vi "Do Critical Stuff.vi"() -> ()   [LabVIEW 2017]
uses:
  <vilib>/userdefined/High Color/nirio_resource_hc.ctl
  <vilib>/LabVIEW Targets/FPGA/cRIO/shared/nicrio_ModuleControls/nicrio_cRIO-9232_ConfigModeRing.ctl
  <vilib>/LabVIEW Targets/FPGA/cRIO/shared/nicrio_ModuleControls/nicrio_cRIO-9230_DataRatesRing2.ctl
  <vilib>/LabVIEW Targets/FPGA/cRIO/shared/nicrio_ModuleControls/nicrio_cRIO-9227_DataRatesRing.ctl
  <vilib>/Platform/TimedLoop/XDataNode/timing_clust.ctl
  <vilib>/Platform/TimedLoop/XDataNode/nitl_modes.ctl
  <vilib>/Platform/TimedLoop/XDataNode/wakeup.ctl
  <vilib>/FPGAPlugInAG/cRIO-9035/niLvFpga_Open_cRIO-9035.vi
  <vilib>/rvi/interface/common/dynamic/niFpgaDynamicAddResources.vi
  <vilib>/FPGAPlugInAG/Dynamic/niLvFpga_Reset_Dynamic.vi
  <vilib>/Utility/error.llb/Error Cluster From Error Code.vi
  <vilib>/rvi/errors/niLvFpgaAdjustHostInterfaceError.vi
  <vilib>/FPGAPlugInAG/Dynamic/niLvFpga_Run_Dynamic.vi
  <vilib>/RVI Host/nirviSupport.llb/nirviErrorClusterFromErrorCode.vi
  <vilib>/LabVIEW Targets/FPGA/RIO/CompactRIO/cRIO-91xx/cRIO-91XX_ReadTEDSImpl.vi
  <vilib>/FPGAPlugInAG/cRIO-9035/niLvFpga_Reset_cRIO-9035.vi
  <vilib>/FPGAPlugInAG/cRIO-9035/niLvFpga_Run_cRIO-9035.vi
  <vilib>/Platform/TimedLoop/XDataNode/loadnilvce.vi
  <vilib>/FPGAPlugInAG/cRIO-9035/niLvFpga_Close_cRIO-9035.vi
  <vilib>/FPGAPlugInAG/Dynamic/niLvFpga_Close_Dynamic.vi
  <vilib>/rvi/interface/nirviOpenFPGA/nirviOpenFPGA.xnode
  FPGA Bitfiles/80Ton_FPGATarget_accelerometer_vQr4SS40msc.lvbitx
  FPGA Bitfiles/accelerometer.vi
  <vilib>/rvi/interface/nirviMethod/nirviMethod.xnode
  <vilib>/rvi/interface/nirviReadWriteControl/nirviReadWriteControl.xnode
  <vilib>/platform/TimedLoop/XDataNode/XDataNode.xnode
  <vilib>/rvi/interface/nirviCloseFPGA/nirviCloseFPGA.xnode
  <vilib>/rvi/interface/nirviMethod/StockFPGA_InlinedMethodWaitForSingleIRQ.vi
  <vilib>/FPGAPlugInAG/Dynamic/niLvFpga_WaitOnIrq_Dynamic.vi
  <vilib>/FPGAPlugInAG/Dynamic/niLvFpga_AcknowledgeIrq_Dynamic.vi
  NiFpgaLv.dll
  <vilib>/rvi/interface/Simulation/niFpgaSimulationCallBeginRW.vi
  <vilib>/Platform/TimedLoop/XDataNode/XDNodeRunTimeDep.lvlib
panel:
  out "Compressor VFD Output Current (A)":dbl
  out "Compressor VFD Output Frequency (Hz)":dbl
  out "Water Pump Frequency (Hz)":dbl
  in  "Are the values not stupid numbers anymore?":bool
  out "Host error out 2":errorcluster
  out "FPGA error out":errorcluster
  out "Elements Remaining 2":u32
  out "Data FIFO Full 2":bool
  in  "Full Open Time":dbl
  out "Waveform Graph 3":dbl[](graph)
  out "loop iter":i32
  out "loopcheck":i32
  out "millisecond timer value 3":u32
  out "millisecond timer value 4":u32
  out "loopcheck 2":i32
  out "100% Open Time 2":dbl
  out "millisecond timer value 5":u32
  out "millisecond timer value 6":u32
  out "millisecond timer value 8":u32
  out "millisecond timer value 7":u32
  out "%oOpen_save":dbl format="%#_13g"
  out "size(s)":i32
  in  "?":bool
  out "Pdis2":dbl
  in  "output cluster":T1
  out "loop iter 4":u32
  out "loop iter 3":u32
  in  "Economizer ?":bool
  out "loop iter 2":i32
  out "x > y?":bool
  out "x .and. y?":bool
  out "Host error out 3":errorcluster
  out "result":bool
  out "FPGA Error Out":errorcluster
  out "Host error out":errorcluster
  in  "Host Loop update rate (ms)":u32=100
  in  "stop":bool
  out "Elements Remaining":u32
  out "Open Loop":bool[](array[boolean])
  out "Short Circuit":bool[](array[boolean])
  out "Data FIFO Full":bool
  out "Waveform Graph":waveform(dbl)[](graph)
  out "Atmospheric Pressure":dbl
  out "element":dbl
  in  "Path 10":path
  in  "Path 9":path
  in  "Path 8":path
  in  "Path 7":path
  in  "Path 6":path
  in  "Path 5":path
  in  "Path 4":path
  in  "Path":path
  in  "Path 2":path
  in  "Path 3":path
  in  "Tab Control":T2(tab)
  in  "Units":string(combo)="IP"
  in  "?":dbl=0.9992
  in  "Tdis":dbl=0.0747
  in  "?":dbl=-0.0246
  in  "Tsuc":dbl=0.998
  in  "?":dbl
  in  "T07":dbl=1.0
  in  "?":dbl=-0.0404
  in  "Tsuc2":dbl=0.9934
  in  "?":dbl=0.0059
  in  "T05":dbl=0.9998
  in  "?":dbl=0.0161
  in  "T04":dbl=1.0002
  in  "?":dbl=0.0174
  in  "Tdis2":dbl=0.9998
  in  "P03":dbl=0.9962
  in  "?":dbl=0.0158
  in  "P04":dbl=0.9943
  in  "?":dbl=-0.8769
  in  "P01":dbl=1.0
  in  "?":dbl
  in  "P02":dbl=1.0
  in  "?":dbl
  in  "P05":dbl=0.9959
  in  "?":dbl=-0.6009
  in  "P06":dbl=0.991
  in  "?":dbl=-0.236
  in  "P07":dbl=1.0
  in  "?":dbl
  in  "P08":dbl=0.9971
  in  "?":dbl=-0.509
  in  "P09":dbl=0.9954
  in  "?":dbl=-0.7109
  in  "Controller Toggle P 2":bool
  in  "Reinitialize Controller P 2":bool
  in  "Current Intermediate P":dbl format="%#_13g"
  in  "Desired Intermediate P":dbl
  in  "Controller Toggle T 2":bool
  in  "Reinitialize Controller T 2":bool
  in  "Current Intermediate T":dbl format="%#_13g"
  in  "Desired Intermediate T":dbl
  in  "?":enum32{"Page 1", "Page 2"}(tab)
  out "Economizer\nFine Liquid Position":dbl(slide) min=0.0 max=100.0 step=1.0 scale=0.0..100.0
  in  "Economizer\nFine Liquid Adjust":dbl(slide) min=0.0 max=100.0 step=1.0 scale=0.0..100.0
  out "Economizer\nLiquid Coarse Position":dbl(slide) min=0.0 max=100.0 step=1.0 scale=0.0..100.0
  in  "Economizer\nLiquid Coarse Adjust":dbl(slide) min=0.0 max=100.0 step=1.0 scale=0.0..100.0
  in  "PID gains in Coarse Liquid":T3
  in  "PID gains in Fine Liquid":T3
  in  "Autotune CoarseLiquid":bool
  in  "Accept Autotune Coarse Liquid":bool
  in  "Autotune Fine Liquid":bool
  in  "Accept Autotune Fine Liquid":bool
  out "PID gains out Coarse Liquid":T3
  out "PID gains out Fine Liquid":T3
  out "tuning completed? Coarse Liquid":bool
  out "tuning completed? Fine Liquid":bool
  in  "?":enum32{"Page 1", "Page 2"}(tab)
  out "Economizer Gas\n Fine Position":dbl(slide) min=0.0 max=100.0 step=1.0 scale=0.0..100.0
  in  "Economizer Gas\n Fine Adjust":dbl(slide) min=0.0 max=100.0 step=1.0 scale=0.0..100.0
  out "Economizer Gas\n Coarse Position":dbl(slide) min=0.0 max=100.0 step=1.0 scale=0.0..100.0
  in  "Economizer Gas\n Coarse Adjust":dbl(slide) min=0.0 max=100.0 step=1.0 scale=0.0..100.0
  in  "PID gains in Coarse gas":T3
  in  "PID gains in Fine Gas":T3
  in  "Autotune Coarse":bool
  in  "Accept Autotune Coarse":bool
  in  "Autotune Fine Gas":bool
  in  "Accept Autotune Fine":bool
  out "PID gains out Coarse Gas":T3
  out "PID gains out Fine Gas":T3
  out "tuning completed? Coarse Gas":bool
  out "tuning completed? Fine Gas":bool
  in  "?":bool
  in  "Reinitialize Controller T":bool
  in  "Delta T Threshold":dbl=5.0 format="%#_13g"
  in  "Tonnage Threshold":dbl=40.0 format="%#_13g"
  in  "Delta P Threshold":dbl=5.0 format="%#_13g"
  in  "Desired Tsuc":dbl
  in  "Desired Psuc":dbl
  in  "Tab Control 3":enum32{"Page 1", "Page 2", "Page 3"}(tab)
  in  "Small Liquid Adjust":dbl(slide) scale=0.0..100.0 scale format="%#_3g"
  in  "Medium Liquid Adjust":dbl(slide) scale=0.0..100.0 scale format="%#_3g"
  in  "Large Liquid Adjust  2":dbl(slide) scale=0.0..100.0 scale format="%#_3g"
  out "Output Large Liq":dbl(slide) scale=0.0..100.0
  out "Output Medium Liq":dbl(slide) scale=0.0..100.0
  out "Output Small Liq":dbl(slide) scale=0.0..100.0
  in  "Accept Autotune Small Liquid":bool
  in  "Autotune Small Liquid":bool
  in  "PID gains in Small Liquid":T3={"proportional gain (Kc)"=-0.0413, "integral time (Ti, min)"=12.063, "derivative time (Td, min)"=0.0}
  in  "PID gains in Medium Liquid":T3={"proportional gain (Kc)"=-0.22, "integral time (Ti, min)"=2.9, "derivative time (Td, min)"=0.0}
  in  "Accept Autotune Medium Liquid":bool
  in  "Autotune Medium Liquid":bool
  in  "PID gains in Large Liquid":T3
  in  "Accept Autotune Large  Liquid":bool
  in  "Autotune Large Liquid":bool
  out "PID gains out Large Liquid":T3
  out "PID gains out Medium Liquid":T3
  out "PID gains out Small Liquid":T3
  out "tuning completed? Large Liq":bool
  out "tuning completed? Medium Liq":bool
  out "tuning completed? Small Liq":bool
  out "Suction Temperature":dbl[][](graph)
  in  "Tab Control 2":enum32{"Page 1", "Page 2", "Page 3"}(tab)
  in  "Large Gas Adjust":dbl(slide) scale=0.0..100.0 scale format="%#_3g"
  in  "Medium Gas Adjust":dbl(slide) scale=0.0..100.0 scale format="%#_3g"
  in  "Small Gas Adjust":dbl(slide) scale=0.0..100.0 scale format="%#_3g"
  out "Output Large Gas":dbl(slide) scale=0.0..100.0
  out "Output Medium Gas":dbl(slide) scale=0.0..100.0
  out "Output Small Gas":dbl(slide) scale=0.0..100.0
  in  "PID gains in Large gas":T3
  in  "PID gains in Medium Gas":T3={"proportional gain (Kc)"=0.542, "integral time (Ti, min)"=2.03, "derivative time (Td, min)"=0.0}
  in  "PID gains in Small Gas":T3={"proportional gain (Kc)"=0.173, "integral time (Ti, min)"=0.636, "derivative time (Td, min)"=0.0}
  in  "Autotune Large":bool
  in  "Accept Autotune Large":bool
  in  "Autotune Medium Gas":bool
  in  "Accept Autotune Medium":bool
  in  "Autotune Small":bool
  in  "Accept Autotune Small":bool
  out "PID gains out Large Gas":T3
  out "PID gains out Medium Gas":T3
  out "PID gains out Small Gas":T3
  out "tuning completed? Large Gas":bool
  out "tuning completed? Medium Gas":bool
  out "tuning completed? Small Gas":bool
  out "Suction Pressure":dbl[][](graph)
  in  "Reinitialize Controller P":bool
  in  "?":bool
  out "Controller Toggle T":bool
  out "Controller Toggle P":bool
  out "Current Tsuc":dbl format="%#.3g"
  out "Current Psuc":dbl format="%#.3g"
  out "Controller Toggle T 3":bool
  out "Controller Toggle P 3":bool
  out "Pdis":dbl format="%#.3g"
  out "element 2":dbl
  out "Tonnage":dbl
  in  "file for water pump 2":path
  in  "Fine slide in P 3":refnum<vi>
  in  "?":enum32{"Page 1", "Page 2", "Page 3"}(tab)
  in  "Coarse Water Adjust":dbl(slide) scale=0.0..100.0 scale format="%#_3g"
  out "Water Valve Output":dbl(slide) scale=0.0..100.0 scale format="%#_3g"
  in  "Fine Water Adjust":dbl(slide) scale=0.0..60.0 scale format="%#_3g"
  out "Water Pump Output":dbl(slide) scale=0.0..60.0 scale format="%#_3g"
  in  "PID gains in Water Valve":T3={"proportional gain (Kc)"=0.081, "integral time (Ti, min)"=6.75, "derivative time (Td, min)"=0.0}
  out "PID gains out Coarse Water":T3
  in  "autotune? Coarse Water":bool
  in  "Accept Autotune Water":bool
  out "tuning completed? Water Valve":bool
  in  "PID gains in water pump 2":T3={"proportional gain (Kc)"=-0.161, "integral time (Ti, min)"=1.936, "derivative time (Td, min)"=0.0}
  out "PID gains out (fine water)":T3
  in  "autotune? water pump 2":bool
  in  "Accept Autotune Water Pump 2":bool
  out "tuning completed? Water Pump":bool
  out "Discharge Pressure":dbl[][](graph)
  in  "file for fine gas":path
  in  "Fine slide in P 2":refnum<vi>
  in  "Desired Pdis":dbl
  in  "Reinitialize Controller":bool
  in  "Controller Toggle P 4":bool
  out "Controller Toggle Water":bool
  in  "Condensing Press Threshold":dbl=5.0 format="%#_13g"
  out "Current Pdis":dbl format="%#.3g"
  in  "Start Water Pump":bool
  in  "Tab Control 4":enum32{"Page 1", "Page 2"}(tab)
  in  "Oil Pump Speed Adjust":dbl(slide) min=0.0 max=100.0 step=1.0 scale=0.0..60.0
  out "Oil Pump Output":dbl(slide) scale=0.0..60.0
  in  "PID gains in oil pump":T3
  out "PID gains out oil pump":T3
  in  "autotune? oil pump":bool
  in  "Accept Autotune Oil Pump":bool
  out "tuning completed?":bool
  in  "Start Oil Pump":bool
  out "Closed":bool
  out "Open":bool
  in  "Timing Complete?":bool
  in  "Open":bool
  in  "Close":bool
  in  "Close 2":bool
  in  "Open 2":bool
  in  "RIO Device 2":T4="RIO0"
  in  "Data Rate 2":T5=25 items=["50.000 kS/s (NI 9227)"=1, "25.000 kS/s (NI 9227)"=2, "16.667 kS/s (NI 9227)"=3, "12.500 kS/s (NI 9227)"=4, "10.000 kS/s (NI 9227)"=5, "8.333 kS/s (NI 9227)"=6, "7.143 kS/s (NI 9227)"=7, "6.250 kS/s (NI 9227)"=8, "5.556 kS/s (NI 9227)"=9, "5.000 kS/s (NI 9227)"=10, "4.545 kS/s (NI 9227)"=11, "4.167 kS/s (NI 9227)"=12, "3.846 kS/s (NI 9227)"=13, "3.571 kS/s (NI 9227)"=14, "3.333 kS/s (NI 9227)"=15, "3.125 kS/s (NI 9227)"=16, "2.941 kS/s (NI 9227)"=17, "2.778 kS/s (NI 9227)"=18, "2.632 kS/s (NI 9227)"=19, "2.500 kS/s (NI 9227)"=20, "2.381 kS/s (NI 9227)"=21, "2.273 kS/s (NI 9227)"=22, "2.174 kS/s (NI 9227)"=23, "2.083 kS/s (NI 9227)"=24, "2.000 kS/s (NI 9227)"=25, "1.923 kS/s (NI 9227)"=26, "1.852 kS/s (NI 9227)"=27, "1.786 kS/s (NI 9227)"=28, "1.724 kS/s (NI 9227)"=29, "1.667 kS/s (NI 9227)"=30, "1.613 kS/s (NI 9227)"=31]
  in  "Host Loop update rate (ms) 2":u32=100
  out "Waveform Graph 2":waveform(dbl)[](graph)
  in  "stop 2":bool
  out "millisecond timer value":u32
  out "100% Open Time":dbl
  out "millisecond timer value 2":u32
  out "%Open":dbl(slide) scale=0.0..100.0
  out "Closed 2":bool
  out "Open  3":bool
  out "Controller Toggle Oil Pump":bool
  in  "Controller Toggle P 8":bool
  in  "Fine slide in P 4":refnum<vi>
  in  "file for oil pump 3":path
  in  "PID gains in water pump":T3
  in  "autotune? water pump":bool
  in  "file for water pump":path
  in  "Fine slide in P":refnum<vi>
  in  "Accept Autotune Water Pump":bool
  in  "Compressor Speed Adjust":dbl(slide) min=0.0 max=100.0 step=1.0 scale=0.0..60.0
  in  "Controller Toggle P 6":bool=TRUE
  out "acceleration v time":waveform(dbl)[](graph)
  in  "RIO Device":T4="RIO0"
  in  "Display TEDS Data":bool
  in  "TEDS Template File Directory":path=path "C:/"
  in  "Input Configuration":T6=2 items=["AC Coupled", "DC Coupled", "IEPE AC Coupled"]
  in  "Data Rate":T7=10 items=["12.800 kS/s (NI 9230)"=10, "11.378 kS/s (NI 9230)"=36, "10.240 kS/s (NI 9230)"=21, "9.309 kS/s (NI 9230)"=44, "8.533 kS/s (NI 9230)"=14, "7.877 kS/s (NI 9230)"=52, "7.314 kS/s (NI 9230)"=29, "6.827 kS/s (NI 9230)"=60, "6.400 kS/s (NI 9230)"=18, "6.024 kS/s (NI 9230)"=68, "5.689 kS/s (NI 9230)"=37, "5.389 kS/s (NI 9230)"=76, "5.120 kS/s (NI 9230)"=22, "4.876 kS/s (NI 9230)"=84, "4.655 kS/s (NI 9230)"=45, "4.452 kS/s (NI 9230)"=92, "4.267 kS/s (NI 9230)"=26, "4.096 kS/s (NI 9230)"=100, "3.938 kS/s (NI 9230)"=53, "3.657 kS/s (NI 9230)"=30, "3.413 kS/s (NI 9230)"=61, "3.200 kS/s (NI 9230)"=34, "3.012 kS/s (NI 9230)"=69, "2.844 kS/s (NI 9230)"=38, "2.695 kS/s (NI 9230)"=77, "2.560 kS/s (NI 9230)"=42, "2.438 kS/s (NI 9230)"=85, "2.327 kS/s (NI 9230)"=46, "2.226 kS/s (NI 9230)"=93, "2.133 kS/s (NI 9230)"=50, "2.048 kS/s (NI 9230)"=101, "1.969 kS/s (NI 9230)"=54, "1.829 kS/s (NI 9230)"=58, "1.707 kS/s (NI 9230)"=62, "1.600 kS/s (NI 9230)"=66, "1.506 kS/s (NI 9230)"=70, "1.422 kS/s (NI 9230)"=74, "1.347 kS/s (NI 9230)"=78, "1.280 kS/s (NI 9230)"=82, "1.219 kS/s (NI 9230)"=86, "1.164 kS/s (NI 9230)"=90, "1.113 kS/s (NI 9230)"=94, "1.067 kS/s (NI 9230)"=98, "1.024 kS/s (NI 9230)"=102, "0.985 kS/s (NI 9230)"=106]
  out "magnitudes":cluster{"f0":dbl, "df":dbl, "magnitude":dbl[]}[](graph)
  out "rotational speed (rpm)":dbl
  out "Compressor Speed (Hz)":dbl
  out "Controller Toggle P 5":bool
  out "Compressor Speed Output":dbl(slide) scale=0.0..60.0
  in  "Start Compressor":bool
  out "Spool x acceleration (Hz)":dbl
  out "Spool y acceleration (Hz)":dbl
  # "Thermocouple Calibration Data"
  # "Pressure Transducer Calibration Data"
  # "Slope"
  # "y-intercept"
  # "Slope"
  # "y-intercept"
  # "Start Up Procedure"
  # "1. Check all safety circuit components to make sure safety loop is closed and VFD's have no faults\n\n2. Check that suction and discharge ball valves are in the open position\n\n3. Put EXV and Oil valves into position\n\n4. Check oil separator sight glass for oil\n\n5. Start cooling water\n\n6. Start compressor"
  # "RTD Calibration Data"
  # "Slope"
  # "y-intercept"
  # "Coarse Water Adjust - Valve"
  # "Fine Water Adjust - Pump"
  # "Oil Pump Speed Control"
  # "Compressor Speed Control"
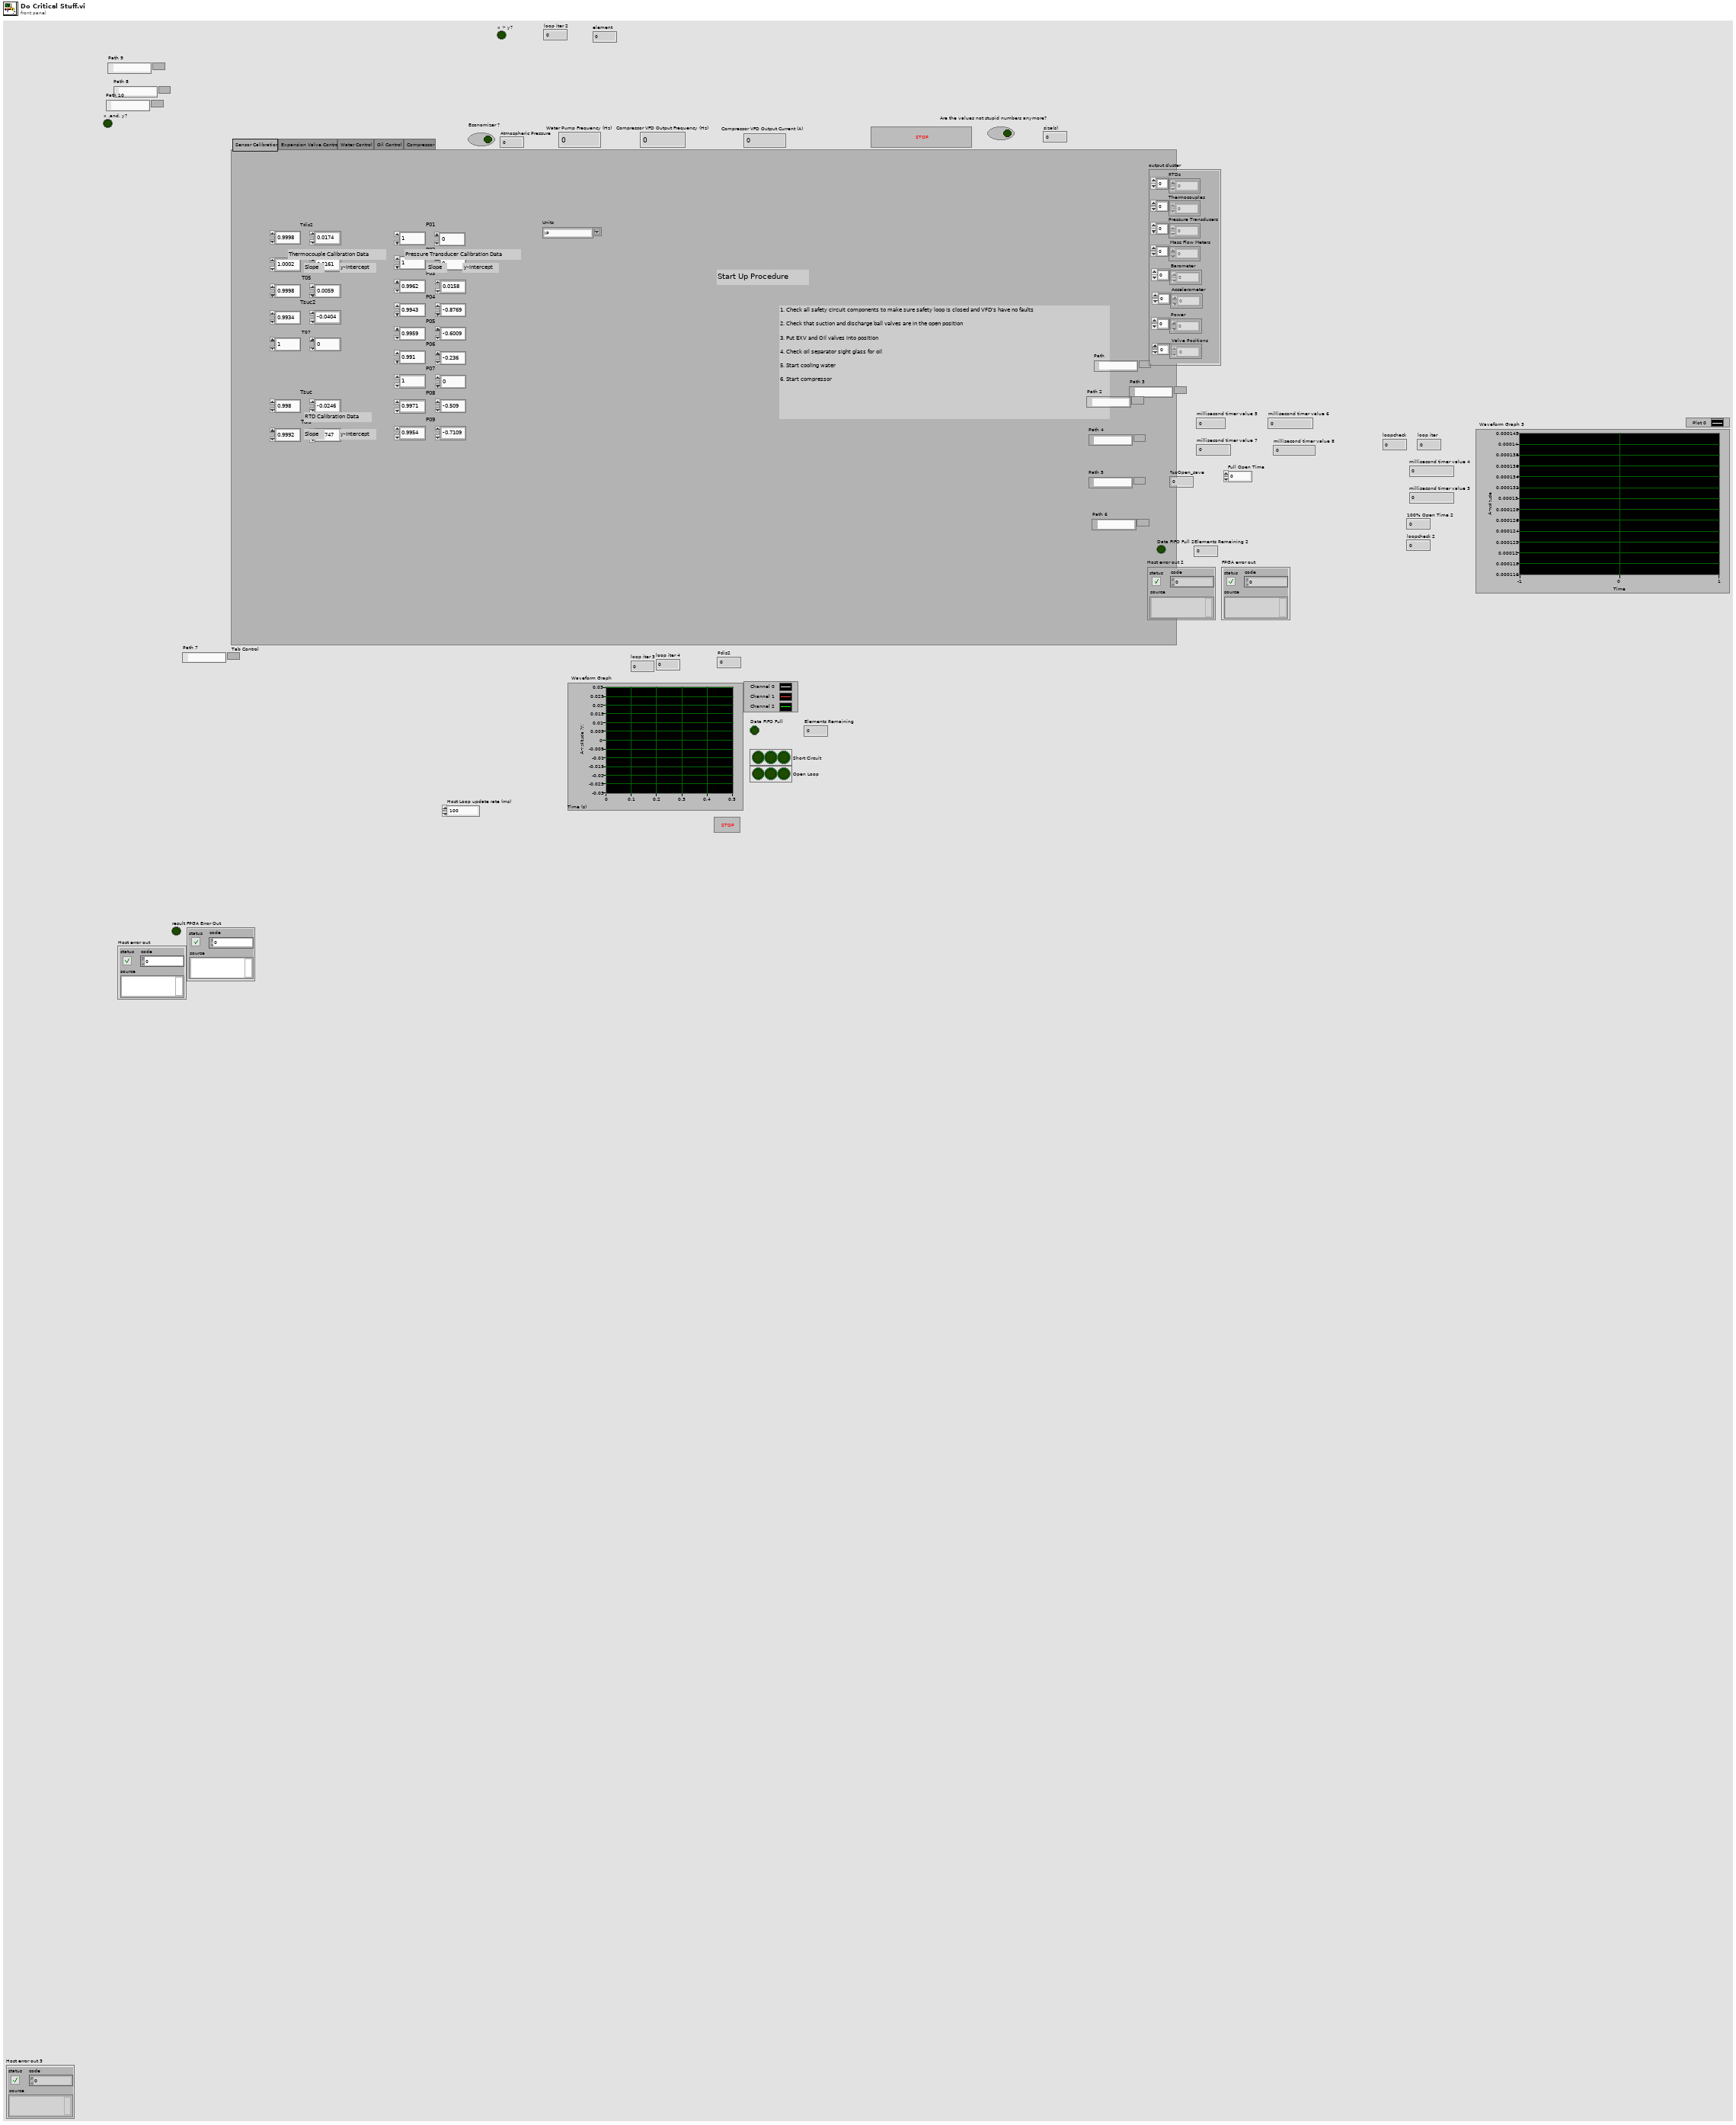
[diagram p1: front panel]
types:
  T1 = cluster{"RTDs":dbl[], "Thermocouples":dbl[], "Pressure Transducers":dbl[], "Mass Flow Meters":dbl[], "Barometer":dbl[], "Accelerometer":dbl[], "Power":dbl[], "Valve Positions":dbl[]}
  T2 = enum32{"Sensor Calibration", "Expansion Valve Control", "Water Control", "Oil Control", "Compressor"}
  T3 = cluster{"proportional gain (Kc)":dbl, "integral time (Ti, min)":dbl, "derivative time (Td, min)":dbl}
  T4 = typedef "nirio_resource_hc.ctl" = tag
  T5 = typedef "nicrio_cRIO-9227_DataRatesRing.ctl" = u8
  T6 = typedef "nicrio_cRIO-9232_ConfigModeRing.ctl" = u8
  T7 = typedef "nicrio_cRIO-9230_DataRatesRing2.ctl" = u8
  T8 = cluster{"TEDS Error?":bool, "TEDS Error":string, "TEDS Data":string[][]}
  T9 = typedef "XDNodeRunTimeDep.lvlib/timing_clust.ctl" = cluster{"Expected End [f-1]":u64, "Actual End [f-1]":u64, "Finished Late? [f-1]":bool, "Expected End [i-1]":u64, "Actual End [i-1]":u64, "Finished Late? [i-1]":bool, "Expected Start [i]":u64, "Actual Start [i]":u64, "Expected Start [f]":u64, "Actual Start [f]":u64, "Source Name":string, "Structure Name":string, "Period":i64, "Deadline":i64, "Offset":i64, "Start":i64, "Priority":i32, "Timeout":i32, "Mode":T10, "Wakeup Reason":T11, "Error":errorcluster, "Source Type":string, "Secondary Source Type":string, "Global End Time":u64, "Global Start Time":u64, "Frame Duration":u64, "Iteration Duration":u64, "Assigned CPU":i32, "I/O Scan Engine Mode":u32}
  T10 = typedef "XDNodeRunTimeDep.lvlib/nitl_modes.ctl" = enum32{"No Change", "Process missed periods, maintain original phase", "Discard missed periods, maintain original phase", "Process missed periods, ignore original phase", "Discard missed periods, ignore original phase"}
  T11 = typedef "XDNodeRunTimeDep.lvlib/wakeup.ctl" = enum32{"Normal", "Aborted", "Asynchronous wakeup", "Timing source error", "Timed loop error", "Timeout"}
  T12 = cluster{"Compressor Speed Adjust":dbl, "autotune? water pump":bool, "Fine slide in P":refnum<vi>, "file for water pump":path, "Accept Autotune Water Pump":bool, "PID gains in water pump":cluster{"proportional gain (Kc)":dbl, "integral time (Ti, min)":dbl, "derivative time (Td, min)":dbl}}
  T13 = cluster{"Oil Pump Speed Adjust":dbl, "autotune? oil pump ":bool, "Fine slide in P 4":refnum<vi>, "file for oil pump 3":path, "Accept Autotune Oil Pump":bool, "PID gains in oil pump ":cluster{"proportional gain (Kc)":dbl, "integral time (Ti, min)":dbl, "derivative time (Td, min)":dbl}}
  T14 = cluster{"output to slide":dbl, "PID gains out":cluster{"proportional gain (Kc)":dbl, "integral time (Ti, min)":dbl, "derivative time (Td, min)":dbl}, "tuning completed?":bool, "Controller Toggle P 2":bool}
  T15 = cluster{"Coarse Water Adjust":dbl, "autotune? Coarse Water":bool, "Fine slide in P 2":refnum<vi>, "file for fine gas":path, "Accept Autotune Water":bool, "PID gains in Water Valve":cluster{"proportional gain (Kc)":dbl, "integral time (Ti, min)":dbl, "derivative time (Td, min)":dbl}}
  T16 = cluster{"Fine Water Adjust":dbl, "autotune? water pump 2":bool, "Fine slide in P 3":refnum<vi>, "file for water pump 2":path, "Accept Autotune Water Pump 2":bool, "PID gains in water pump 2":cluster{"proportional gain (Kc)":dbl, "integral time (Ti, min)":dbl, "derivative time (Td, min)":dbl}}
  T17 = cluster{"output to slide":dbl, "PID gains out":cluster{"proportional gain (Kc)":dbl, "integral time (Ti, min)":dbl, "derivative time (Td, min)":dbl}, "tuning completed?":bool, "output to slide":dbl, "PID gains out":cluster{"proportional gain (Kc)":dbl, "integral time (Ti, min)":dbl, "derivative time (Td, min)":dbl}, "tuning completed?":bool, "Controller Toggle P 2":bool, bool}
  T18 = cluster{"Economizer Gas\n Coarse Adjust":dbl, "Accept Autotune Coarse":bool, "Economizer Gas\n Coarse Adjust":refnum<vi>, "Path 7":path, "Autotune Coarse":bool, "PID gains in Coarse gas ":cluster{"proportional gain (Kc)":dbl, "integral time (Ti, min)":dbl, "derivative time (Td, min)":dbl}}
  T19 = cluster{"Economizer Gas\n Fine Adjust":dbl, "Accept Autotune Fine":bool, "Economizer Gas\n Fine Adjust":refnum<vi>, "Path 8":path, "Autotune Fine Gas ":bool, "PID gains in Fine Gas":cluster{"proportional gain (Kc)":dbl, "integral time (Ti, min)":dbl, "derivative time (Td, min)":dbl}}
  T20 = cluster{"Economizer\nLiquid Coarse Adjust":dbl, "Accept Autotune Coarse Liquid":bool, "Economizer\nLiquid Coarse Adjust":refnum<vi>, "Path 9":path, "Autotune CoarseLiquid":bool, "PID gains in Coarse Liquid":cluster{"proportional gain (Kc)":dbl, "integral time (Ti, min)":dbl, "derivative time (Td, min)":dbl}}
  T21 = cluster{"Economizer\nFine Liquid Adjust":dbl, "Accept Autotune Fine Liquid":bool, "Economizer\nFine Liquid Adjust":refnum<vi>, "Path 10":path, "Autotune Fine Liquid":bool, "PID gains in Fine Liquid":cluster{"proportional gain (Kc)":dbl, "integral time (Ti, min)":dbl, "derivative time (Td, min)":dbl}}
  T22 = cluster{"Hot Gas Bypass\n Fine Position":dbl, "PID gains out fine gas":cluster{"proportional gain (Kc)":dbl, "integral time (Ti, min)":dbl, "derivative time (Td, min)":dbl}, "tuning completed? fine gas":bool, "Hot Gas Bypass\n Coarse Position":dbl, "PID gains out coarse gas":cluster{"proportional gain (Kc)":dbl, "integral time (Ti, min)":dbl, "derivative time (Td, min)":dbl}, "tuning completed? coarse gas":bool, "P Indicator":bool}
  T23 = cluster{"Liquid\n Fine Position":dbl, "PID gains out fine liq":cluster{"proportional gain (Kc)":dbl, "integral time (Ti, min)":dbl, "derivative time (Td, min)":dbl}, "tuning completed? fine liq":bool, "Liquid\n Coarse Position":dbl, "PID gains out coarse liq":cluster{"proportional gain (Kc)":dbl, "integral time (Ti, min)":dbl, "derivative time (Td, min)":dbl}, "tuning completed? coarse liq":bool, "T Indicator":bool}
  T24 = cluster{"Large Gas Adjust ":dbl, "Autotune Large":bool, "Path":path, "Large Gas Adjust ":refnum<vi>, "Accept Autotune Large ":bool, "PID gains in Large gas":cluster{"proportional gain (Kc)":dbl, "integral time (Ti, min)":dbl, "derivative time (Td, min)":dbl}}
  T25 = cluster{"Medium Gas Adjust":dbl, "Autotune Medium Gas":bool, "Path 2":path, "Medium Gas Adjust":refnum<vi>, "Accept Autotune Medium":bool, "PID gains in Medium Gas":cluster{"proportional gain (Kc)":dbl, "integral time (Ti, min)":dbl, "derivative time (Td, min)":dbl}}
  T26 = cluster{"Small Gas Adjust":dbl, "Autotune Small":bool, "Path 3":path, "Small Gas Adjust":refnum<vi>, "Accept Autotune Small":bool, "PID gains in Small Gas ":cluster{"proportional gain (Kc)":dbl, "integral time (Ti, min)":dbl, "derivative time (Td, min)":dbl}}
  T27 = cluster{"Large Liquid Adjust  2":dbl, "Autotune Large Liquid":bool, "Path 4":path, "Large Liquid Adjust  2":refnum<vi>, "Accept Autotune Large  Liquid":bool, "PID gains in Large Liquid":cluster{"proportional gain (Kc)":dbl, "integral time (Ti, min)":dbl, "derivative time (Td, min)":dbl}}
  T28 = cluster{"Medium Liquid Adjust":dbl, "Autotune Medium Liquid":bool, "Path 5":path, "Medium Liquid Adjust":refnum<vi>, "Accept Autotune Medium Liquid":bool, "PID gains in Medium Liquid":cluster{"proportional gain (Kc)":dbl, "integral time (Ti, min)":dbl, "derivative time (Td, min)":dbl}}
  T29 = cluster{"Small Liquid Adjust ":dbl, "Autotune Small Liquid":bool, "Path 6":path, "Small Liquid Adjust ":refnum<vi>, "Accept Autotune Small Liquid":bool, "PID gains in Small Liquid":cluster{"proportional gain (Kc)":dbl, "integral time (Ti, min)":dbl, "derivative time (Td, min)":dbl}}
  T30 = cluster{"output to slide":dbl, "PID gains out":cluster{"proportional gain (Kc)":dbl, "integral time (Ti, min)":dbl, "derivative time (Td, min)":dbl}, "tuning completed?":bool, "output to slide":dbl, "PID gains out":cluster{"proportional gain (Kc)":dbl, "integral time (Ti, min)":dbl, "derivative time (Td, min)":dbl}, "tuning completed?":bool, "output to slide":dbl, "PID gains out":cluster{"proportional gain (Kc)":dbl, "integral time (Ti, min)":dbl, "derivative time (Td, min)":dbl}, "tuning completed?":bool, "Controller Toggle P":bool, bool, bool}
  T31 = cluster{"output to slide":dbl, "PID gains out":cluster{"proportional gain (Kc)":dbl, "integral time (Ti, min)":dbl, "derivative time (Td, min)":dbl}, "tuning completed?":bool, "output to slide":dbl, "PID gains out":cluster{"proportional gain (Kc)":dbl, "integral time (Ti, min)":dbl, "derivative time (Td, min)":dbl}, "tuning completed?":bool, "output to slide":dbl, "PID gains out":cluster{"proportional gain (Kc)":dbl, "integral time (Ti, min)":dbl, "derivative time (Td, min)":dbl}, "tuning completed?":bool, "Controller Toggle T":bool, bool, bool}
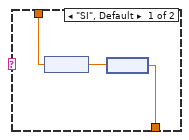
[diagram p5: hidden frame]
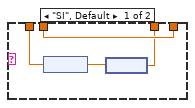
[diagram p6: hidden frame]
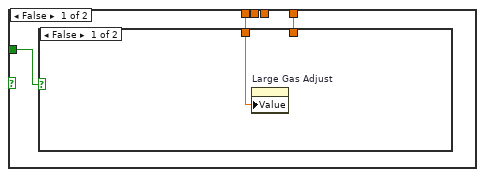
[diagram p8: hidden frame]
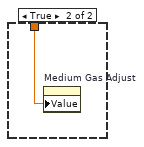
[diagram p9: hidden frame]
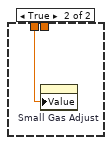
[diagram p10: hidden frame]
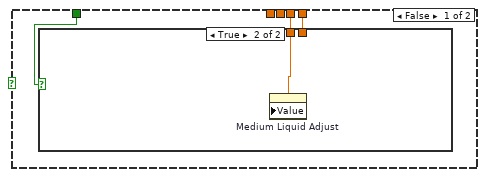
[diagram p12: hidden frame]
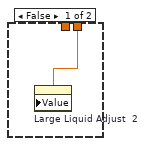
[diagram p13: hidden frame]
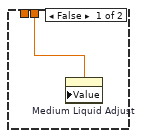
[diagram p14: hidden frame]
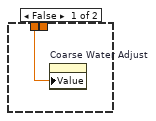
[diagram p16: hidden frame]
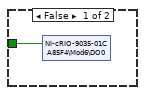
[diagram p19: hidden frame]
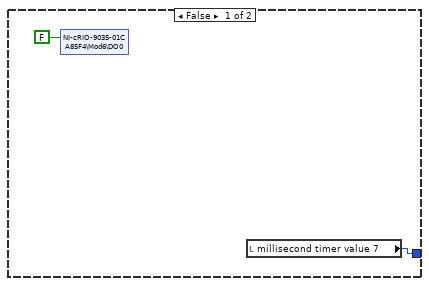
[diagram p20: hidden frame]
diagram:
  w9 = u32 0 ("loop iter 3")
  w10 = u32 0 ("millisecond timer value")
  # "Set up FPGA target"
  n1 = shared-variable "NI-cRIO-9035-01CA85F4\\Untitled Library 2.lvlib\\Data"(dbl[] [] ("Data")) -> ()  [unwired: 1 in, 1 out]
  n2 = xnode "Open FPGA VI Reference"("resource name"="RIO Device") -> ("FPGA VI Reference Out"=w40:refnum<k20>, "error out"=w44:errorcluster)  [unwired: 1 in]
  n3 = xnode "Invoke Method"("FPGA VI Reference In"=w40, "error in"=w44) -> ("FPGA VI Reference Out"=w39:refnum<k20>, "error out"=w41:errorcluster)
  n4 = xnode "Read/Write Control"("FPGA VI Reference In"=w39, "error in"=w41, "Data Rate"="Data Rate", "Input Configuration"="Input Configuration") -> ("FPGA VI Reference Out"=w46:refnum<k20>, "error out"=w45:errorcluster)
  n5 = xnode "Invoke Method"("FPGA VI Reference In"=w46, "error in"=w45) -> ("FPGA VI Reference Out"=w25:refnum<k20>, "error out"=w23:errorcluster)  [unwired: 1 in]
  n6 = xnode "Invoke Method"("FPGA VI Reference In"=w25, "error in"=w23, "IRQ Number(s)"=0, "Timeout (ms)"=15000) -> ("FPGA VI Reference Out"=w24:refnum<k20>, "error out"=w22:errorcluster, "IRQ(s) Asserted"=w16:i32)  [unwired: 1 out]
  n7 = case shown="False" "Display TEDS Data" {
    tunnel: w24 -> [w75 w81]
    tunnel: [w75 w80] -> w18
    tunnel: w22 -> [w74 w79]
    tunnel: [w74 w76] -> w19
    frame False {
    }
    frame True {
      n8 = for {
        N: 3 -> [_]
        tunnel: w81 -> [w92]
        tunnel: [w91] -> w80
        tunnel: [w86] -> w77 mode=indexing
        shift-right: [w87] -> w76
        shift-left: w79 -> [w90]
        i -> [w85]
        n9 = xnode "Invoke Method"("FPGA VI Reference In"=w92, "error in"=w90, "Slot"=1, "Channel"=w85) -> ("FPGA VI Reference Out"=w91:refnum<k20>, "error out"=w88:errorcluster, "TEDS Binary"=w83:bool[], "v0.9 (TEDS)"=w84:bool)
        n10 = call "TEDS Binary to Table.vi"("error in"=w88, "v0.9 TEDS (F)"=w84, "template file directory"="TEDS Template File Directory", "TEDS Binary"=w83) -> ("error out"=w87:errorcluster, "TEDS"=w86:T8)  [unwired: 1 out]
      }
      n11 = call "Display TEDS Data.vi"("TEDS Array"=w77) -> ()  [unwired: 4 out]
    }
  }
  n12 = xnode "Open FPGA VI Reference"("resource name"="RIO Device 2") -> ("FPGA VI Reference Out"=w32:refnum<k20>, "error out"=w29:errorcluster)  [unwired: 1 in]
  n13 = xnode "Invoke Method"("FPGA VI Reference In"=w32, "error in"=w29) -> ("FPGA VI Reference Out"=w31:refnum<k20>, "error out"=w30:errorcluster)
  n14 = local write "%Open"(0.0 ("%Open")) -> ()
  n15 = xnode "Read/Write Control"("FPGA VI Reference In"=w31, "error in"=w30, "Data Rate"="Data Rate 2") -> ("FPGA VI Reference Out"=w27:refnum<k20>, "error out"=w28:errorcluster)
  n16 = xnode "Invoke Method"("FPGA VI Reference In"=w27, "error in"=w28) -> ("FPGA VI Reference Out"=w15:refnum<k20>, "error out"=w7:errorcluster)  [unwired: 1 in]
  n17 = Initialize Array(0.0 ("element"), 0 ("dimension size")) -> (w34:dbl[])
  n18 = Initialize Array(0.0 ("element"), 0 ("dimension size")) -> (w70:dbl[])
  n19 = xnode "Invoke Method"("FPGA VI Reference In"=w18, "error in"=w19, "IRQ Number(s)"=w16) -> ("FPGA VI Reference Out"=w6:refnum<k20>, "error out"=w17:errorcluster)
  n20 = Initialize Array(0.0 ("element"), 0 ("dimension size")) -> (w35:dbl[])
  n21 = Initialize Array(0.0 ("element"), 0 ("dimension size")) -> (w58:dbl[])
  n22 = Initialize Array(0.0 ("element"), 0 ("dimension size")) -> (w55:dbl[])
  n23 = Initialize Array(0.0 ("element"), 0 ("dimension size")) -> (w48:dbl[])
  n24 = node-c288() -> (w5:T9)  [unwired: 4 in]
  n25 = Initialize Array(0.0 ("element"), 0 ("dimension size")) -> (w1:dbl[])
  n26 = timed-loop {
    tunnel: "output cluster" -> [w333]
    tunnel: "Reinitialize Controller P" -> [w463]
    tunnel: "Reinitialize Controller T" -> [w462]
    tunnel: "Delta T Threshold" -> [w460]
    tunnel: "Tonnage Threshold" -> [w461]
    tunnel: "Delta P Threshold" -> [w459]
    tunnel: w70 -> [w445]
    tunnel: w58 -> [w444]
    tunnel: w34 -> [w327]
    tunnel: w55 -> [w443]
    tunnel: "Reinitialize Controller P 2" -> [w372]
    tunnel: "Reinitialize Controller T 2" -> [w371]
    tunnel: w48 -> [w350]
    tunnel: w6 -> [w346]
    tunnel: w17 -> [w345]
    tunnel: [w344] -> w26
    tunnel: [w343] -> w67
    tunnel: [w335] -> w65
    tunnel: w35 -> [w330]
    tunnel: w15 -> [w319]
    tunnel: w7 -> [w318]
    tunnel: [w317] -> w13
    tunnel: [w316] -> w12
    timing: w5 -> [_]
    timing-out: [_] -> w4
    tunnel: w1 -> [w189]
    i -> [w303]
    stop <- w191 stop-if-true
    w145 = 0.5 ("y")
    w150 = 0.2 ("y")
    # "Oil Pump Speed Control"
    # "Compressor Speed Control"
    # "Cooling Water Control"
    # "Bypass Valve Control"
    # "Accelerometer data collection"
    # "Economizer Expansion Valves"
    # "oil valves timing and control"
    # "Create arrays of data from channels"
    # "valve limit - LRA or turned off"
    # "valve moving"
    # "valve limit - LRA or turned off"
    # "valve moving"
    n27 = node-c288() -> ()  [unwired: 1 in, 1 out]
    n28 = control-ref of="Data Rate 2"() -> (w321:refnum<vi>)
    n29 = call "OilValveTiming.vi"("FPGA VI Reference In"=w319, "reference"=w321, "host loop update rate"="Host Loop update rate (ms) 2", "error in"=w318, "stop in"="stop 2") -> ("Waveform Graph"=→"Waveform Graph 3":dbl[], "x > y?"=w222:bool, "x .and. y?"=w298:bool, "Elements Remaining 2"=→"Elements Remaining 2":u32, "FPGA VI Reference Out"=w316:refnum<k20>, "Waveform Graph 2"=→"Waveform Graph 2":waveform(dbl)[], "Data FIFO Full 2"=→"Data FIFO Full 2":bool, "x .and. y? 2"=w285:bool, "x > y? 2"=w216:bool, "Host error out 2"=→"Host error out 2":errorcluster, "error out"=w317:errorcluster)  [unwired: 4 in]
    "x .and. y?" <- w298
    "x > y?" <- w222
    n30 = shared-variable "NI-cRIO-9035-01CA85F4\\Mod6\\DO6"("Start Oil Pump") -> ()  [unwired: 1 in, 1 out]
    n31 = shared-variable "NI-cRIO-9035-01CA85F4\\Mod6\\DO5"("Start Compressor") -> ()  [unwired: 1 in, 1 out]
    n32 = shared-variable "NI-cRIO-9035-01CA85F4\\Mod6\\DO4"("Start Water Pump") -> ()  [unwired: 1 in, 1 out]
    n33 = property on="loop iter 2" class="DigNum (strict)"() -> ("Value"=w284:i32)  [unwired: 2 in, 2 out]
    n34 = And(x=w222, y="Open") -> (x .and. y?=→"Open":bool)
    n35 = property on="loop iter" class="DigNum (strict)"() -> ("Value"=w300:i32)  [unwired: 2 in, 2 out]
    n36 = Equal?(x=w284, y=2.0) -> (x = y?=w287:bool)
    n37 = And(x=w216, y="Open 2") -> (x .and. y?=→"Open  3":bool)
    n38 = shared-variable "NI-cRIO-9035-01CA85F4\\Mod6\\DO2"("Close 2") -> ()  [unwired: 1 in, 1 out]
    n39 = shared-variable "NI-cRIO-9035-01CA85F4\\Mod6\\DO3"("Open 2") -> ()  [unwired: 1 in, 1 out]
    n40 = Equal?(x=0, y=w303) -> (x = y?=w301:bool)
    n41 = case shown="True" w287 {
      tunnel: w284 -> [w601 w603]
      tunnel: [w601 w602] -> w286
      frame False {
      }
      frame True {
        w602 = 0
        # "reset loop iter so process can start again"
        n42 = local read "millisecond timer value 3"() -> (w604:u32)
        n43 = local read "millisecond timer value 4"() -> (w605:u32)
        n44 = Subtract(x=w604, y=w605) -> (x-y=w607:u32)
        n45 = property on="loop iter 2" class="DigNum (strict)"("Value"=w602) -> ()  [unwired: 2 in, 2 out]
        n46 = Divide(x=w607, y=u32 1000) -> (x/y=→"100% Open Time 2":dbl)
        "loopcheck 2" <- w603
      }
    }
    n47 = shared-variable "NI-cRIO-9035-01CA85F4\\Capacity.lvlib\\Capacity"() -> (w281:dbl)  [unwired: 1 in, 1 out]
    n48 = And(x=w216, y="Close 2") -> (x .and. y?=→"Closed 2":bool)
    n49 = case shown="True" w301 {
      frame False {
      }
      frame True {
        n50 = property on="loop iter" class="DigNum (strict)"("Value"=0) -> ()  [unwired: 2 in, 2 out]
      }
    }
    n51 = Equal?(x=w300, y=2.0) -> (x = y?=w304:bool)
    n52 = And(x=w222, y="Close") -> (x .and. y?=→"Closed":bool)
    n53 = case shown="True" "Timing Complete?" {
      tunnel: "Open" -> [w565 w569]
      tunnel: "Full Open Time" -> [_ w568]
      frame False {
        n54 = shared-variable "NI-cRIO-9035-01CA85F4\\Mod6\\DO1"(w565) -> ()  [unwired: 1 in, 1 out]
      }
      frame True {
        n55 = property on="loop iter 3" class="DigNum (strict)"() -> ("Value"=w570:u32)  [unwired: 2 in, 2 out]
        n56 = feedback #1() -> (w566:dbl)  [unwired: 1 in]
        "%oOpen_save" <- w566
        n57 = Equal?(x=w570, y=u32 0) -> (x = y?=w571:bool)
        n58 = case shown="True" w569 {
          tunnel: w571 -> [_ w584]
          tunnel: w570 -> [_ w585]
          tunnel: w569 -> [_ w582]
          tunnel: w568 -> [_ w578]
          tunnel: [w573 _] -> w567
          tunnel: w566 -> [_ w576]
          frame False {
            n59 = shared-variable "NI-cRIO-9035-01CA85F4\\Mod6\\DO1"(FALSE ("DO1")) -> ()  [unwired: 1 in, 1 out]
            n60 = property on="loop iter 3" class="DigNum (strict)"("Value"=u32 0 ("loop iter 3")) -> ()  [unwired: 2 in, 2 out]
            n61 = local read "%Open"() -> (w573:dbl)
          }
          frame True {
            n62 = property on="loop iter 3" class="DigNum (strict)"() -> ("Value"=w579:u32)  [unwired: 2 in, 2 out]
            n63 = And(x=w582, y=w584) -> (x .and. y?=w583:bool)
            n64 = shared-variable "NI-cRIO-9035-01CA85F4\\Mod6\\DO1"(TRUE) -> ()  [unwired: 1 in, 1 out]
            n65 = case shown="True" w583 {
              tunnel: w585 -> [_ w600]
              frame False {
              }
              frame True {
                n66 = Increment(x=w600) -> (x+1=w598:u32)
                n67 = Tick Count (ms)() -> (millisecond timer value=→"millisecond timer value 6":u32)
                n68 = property on="loop iter 3" class="DigNum (strict)"("Value"=w598) -> ()  [unwired: 2 in, 2 out]
              }
            }
            n69 = Equal?(x=w579, y=u32 1) -> (x = y?=w581:bool)
            n70 = Tick Count (ms)() -> (millisecond timer value=w577:u32)
            "millisecond timer value 5" <- w577
            n71 = case shown="True" w581 {
              tunnel: w577 -> [_ w593]
              tunnel: w578 -> [_ w590]
              tunnel: w576 -> [_ w589]
              frame False {
                (unwired) 0.0
              }
              frame True {
                n72 = local read "millisecond timer value 6"() -> (w592:u32)
                n73 = Multiply(x=w590, y=1000.0) -> (x*y=w597:dbl)
                n74 = Subtract(x=w593, y=w592) -> (x-y=w591:u32)
                n75 = Divide(x=w591, y=w597) -> (x/y=w594:dbl)
                n76 = Multiply(x=w594, y=100.0) -> (x*y=w588:dbl)
                n77 = Add(x=w589, y=w588) -> (x+y=→"%Open":dbl)
              }
            }
          }
        }
        n78 = feedback-in #1(w567) -> ()
      }
    }
    n79 = case shown="True" w304 {
      tunnel: w300 -> [w615 w618]
      tunnel: [w615 w617] -> w299
      frame False {
      }
      frame True {
        w617 = 0
        # "reset loop iter so process can start again"
        n80 = local read "millisecond timer value 2"() -> (w619:u32)
        n81 = local read "millisecond timer value"() -> (w620:u32)
        n82 = property on="loop iter" class="DigNum (strict)"("Value"=w617) -> ()  [unwired: 2 in, 2 out]
        n83 = Subtract(x=w619, y=w620) -> (x-y=w621:u32)
        n84 = Divide(x=w621, y=u32 1000) -> (x/y=→"100% Open Time":dbl)
        "loopcheck" <- w618
      }
    }
    n85 = case shown="True" "Timing Complete?" {
      tunnel: "Close" -> [w550 w555]
      tunnel: [_ w551] -> w260
      frame False {
        n86 = shared-variable "NI-cRIO-9035-01CA85F4\\Mod6\\DO0"(w550) -> ()  [unwired: 1 in, 1 out]
      }
      frame True {
        n87 = property on="loop iter 4" class="DigNum (strict)"() -> ("Value"=w552:u32)  [unwired: 2 in, 2 out]
        n88 = Equal?(x=w552, y=u32 0) -> (x = y?=w553:bool)
        n89 = case shown="True" w555 {
          tunnel: w553 -> [_ w560]
          tunnel: w552 -> [_ w559]
          tunnel: [w556 w558] -> w551
          frame False {
            n90 = shared-variable "NI-cRIO-9035-01CA85F4\\Mod6\\DO0"(FALSE ("DO0")) -> ()  [unwired: 1 in, 1 out]
            n91 = local read "millisecond timer value 7"() -> (w556:u32)
          }
          frame True {
            n92 = case shown="True" w560 {
              tunnel: w559 -> [_ w564]
              frame False {
              }
              frame True {
                n93 = Increment(x=w564) -> (x+1=w563:u32)
                n94 = Tick Count (ms)() -> (millisecond timer value=→"millisecond timer value 8":u32)
                n95 = property on="loop iter 4" class="DigNum (strict)"("Value"=w563) -> ()  [unwired: 2 in, 2 out]
              }
            }
            n96 = shared-variable "NI-cRIO-9035-01CA85F4\\Mod6\\DO0"(TRUE ("DO0")) -> ()  [unwired: 1 in, 1 out]
            n97 = Tick Count (ms)() -> (millisecond timer value=w558:u32)
            "millisecond timer value 7" <- w558
          }
        }
      }
    }
    n98 = local read "Spool y acceleration (Hz)"() -> (w94:dbl)
    n99 = Divide(x=w281, y=3.517) -> (x/y=w282:dbl)
    "Tonnage" <- w282
    n100 = local read "Spool x acceleration (Hz)"() -> (w95:dbl)
    n101 = Equal?(x=w286, y=0.0) -> (x = y?=w296:bool)
    n102 = And(x=w216, y=w296) -> (x .and. y?=w295:bool)
    n103 = local read "Compressor Speed (Hz)"() -> (w329:dbl)
    n104 = case shown="True" w295 {
      tunnel: w286 -> [_ w610]
      frame False {
      }
      frame True {
        n105 = Tick Count (ms)() -> (millisecond timer value=→"millisecond timer value 4":u32)
        n106 = Increment(x=w610) -> (x+1=w609:i32)
        n107 = property on="loop iter 2" class="DigNum (strict)"("Value"=w609) -> ()  [unwired: 2 in, 2 out]
      }
    }
    n108 = call "Watt Transducer.vi"("Array in"=w189) -> ("Array out"=w188:dbl[])  [unwired: 10 in]
    n109 = Insert Into Array(array=w330, new element #1=w329, new element #2=w95, new element #3=w94) -> (w328:dbl[])  [unwired: 1 in]
    n110 = call "RTDRead.vi"("Numeric 15"="?", "Numeric 14"="Tdis", "Numeric 13"="?", "Numeric 12"="Tsuc", "Array in"=w445) -> ("Array out"=w464:dbl[])  [unwired: 6 in]
    n111 = call "Mass Flow Meters.vi"("Array in"=w443) -> ("Array out"=w446:dbl[])  [unwired: 10 in]
    n112 = call "ThermocoupleRead.vi"("Array in"=w444, "Numeric 8"="Tsuc2", "Numeric 9"="?", "Numeric 3"="?", "Numeric 2"="Tdis2", "Numeric 4"="T04", "Numeric 5"="?", "Numeric 6"="T05", "Numeric 7"="?", "Numeric 10"="T07", "Numeric 11"="?") -> ("Array out"=w466:dbl[])  [unwired: 4 in]
    n113 = call "barometer.vi"("Array in"=w350) -> ("Array out"=w349:dbl[])  [unwired: 10 in]
    n114 = Greater?(x=w286, y=0.0) -> (0:w291:bool)
    n115 = local read "Units"() -> (w107:string)
    n116 = Not Or(1:w216, 2:w285) -> (0:w289:bool)
    n117 = Index Array(array=w464) -> (element #1=w106:dbl)  [unwired: 3 in, 2 out]
    n118 = Index Array(array=w349) -> (element=w214:dbl)  [unwired: 1 in]
    "Atmospheric Pressure" <- w214
    n119 = call "PTRead.vi"("Array in"=w327, "P06"="P06", "P03"="P03", "P06 1"="?", "P03 1"="?", "P07"="P07", "P04"="P04", "P07 1"="?", "P01"="P01", "P08"="P08", "P01 1"="?", "P04 1"="?", "P02"="P02", "P08 1"="?", "P02 1"="?", "P09"="P09", "P05"="P05", "P09 1"="?", "P05 1"="?", "atm"=w214) -> ("Array out"=w465:dbl[])  [unwired: 7 in]
    n120 = Index Array(array=w465, index #5=4 ("index"), index #6=5 ("index")) -> (element #1=w160:dbl, element #2=w109:dbl, element #3=→"Pdis2":dbl, element #6=→"element 2":dbl)  [unwired: 7 in, 5 out]
    "Current Psuc" <- w160
    n121 = And(x=w285, y=w291) -> (x .and. y?=w293:bool)
    n122 = Index Array(array=w446, index #1=0 ("index")) -> (element #1=→"element":dbl)  [unwired: 1 in, 1 out]
    n123 = And(x=w289, y=w291) -> (x .and. y?=w290:bool)
    n124 = case shown="\"SI\", Default" w107 {
      tunnel: [w472 w474] -> w108
      tunnel: w109 -> [w471 w474]
      frame "SI", Default {
        n125 = node(w471) -> (w473:dbl[unit])
        n126 = node(w473) -> (w472:dbl)
      }
      frame "IP" {
      }
    }
    "Pdis" <- w108
    n127 = Or(x=w290, y=w293) -> (x .or. y?=w292:bool)
    n128 = case shown="True" w292 {
      frame False {
      }
      frame True {
        n129 = Tick Count (ms)() -> (millisecond timer value=→"millisecond timer value 3":u32)
        n130 = property on="loop iter 2" class="DigNum (strict)"("Value"=2) -> ()  [unwired: 2 in, 2 out]
      }
    }
    n131 = local read "Units"() -> (w105:string)
    n132 = case shown="\"IP\", Default" w105 {
      tunnel: [w468 w470] -> w104
      tunnel: w106 -> [w467 w470]
      frame "IP", Default {
        n133 = node(w467) -> (w469:dbl[unit])
        n134 = node(w469) -> (w468:dbl)
      }
      frame "SI" {
      }
    }
    "Current Tsuc" <- w104
    n135 = local read "Desired Pdis"() -> (w146:dbl)
    n136 = local read "Desired Psuc"() -> (w155:dbl)
    n137 = local read "Desired Tsuc"() -> (w151:dbl)
    n138 = Add(x=w146, y=w145) -> (x+y=w144:dbl)
    n139 = Subtract(x=w146, y=w145) -> (x-y=w143:dbl)
    n140 = Build Array(w108, w146, w144, w143) -> (w142:dbl[])
    n141 = Add(x=w151, y=w150) -> (x+y=w152:dbl)
    n142 = Subtract(x=w151, y=w150) -> (x-y=w149:dbl)
    n143 = Add(x=w155, y=0.5) -> (x+y=w156:dbl)
    n144 = Subtract(x=w155, y=0.5) -> (x-y=w153:dbl)
    n145 = Build Array(w104, w151, w152, w149) -> (w148:dbl[])
    n146 = Build Array(w160, w155, w156, w153) -> (w159:dbl[])
    n147 = Build Array(w142) -> (→"Discharge Pressure":dbl[][])
    n148 = call "VFD Feedback.vi"() -> ("Compressor VFD Output Current (A)"=→"Compressor VFD Output Current (A)":dbl, "Compressor VFD Output Frequency (Hz)"=→"Compressor VFD Output Frequency (Hz)":dbl, "Water Pump Frequency (Hz)"=→"Water Pump Frequency (Hz)":dbl)  [unwired: 9 in]
    n149 = Build Array(w148) -> (→"Suction Temperature":dbl[][])
    n150 = Build Array(w159) -> (→"Suction Pressure":dbl[][])
    n151 = property on="loop iter 4" class="DigNum (strict)"() -> ("Value"=w263:u32)  [unwired: 2 in, 2 out]
    n152 = Bundle("Compressor Speed Adjust"="Compressor Speed Adjust", "autotune? water pump"="autotune? water pump", "Fine slide in P"="Fine slide in P", "file for water pump"="file for water pump", "Accept Autotune Water Pump"="Accept Autotune Water Pump", "PID gains in water pump"="PID gains in water pump") -> (w209:T12)  [unwired: 1 in]
    n153 = Equal?(x=w299, y=0.0) -> (x = y?=w313:bool)
    n154 = Greater?(x=w299, y=0.0) -> (0:w308:bool)
    n155 = Equal?(x=w263, y=u32 1) -> (x = y?=w261:bool)
    n156 = Not Or(1:w298, 2:w222) -> (0:w306:bool)
    n157 = case shown="True" w261 {
      tunnel: w260 -> [_ w548]
      tunnel: "Full Open Time" -> [_ w546]
      frame False {
      }
      frame True {
        n158 = Multiply(x=w546, y=1000.0) -> (x*y=w543:dbl)
        n159 = local read "millisecond timer value 8"() -> (w549:u32)
        n160 = Subtract(x=w548, y=w549) -> (x-y=w542:u32)
        n161 = Divide(x=w542, y=w543) -> (x/y=w544:dbl)
        n162 = local read "%Open"() -> (w540:dbl)
        n163 = Multiply(x=w544, y=100.0) -> (x*y=w541:dbl)
        n164 = Subtract(x=w540, y=w541) -> (x-y=w539:dbl)
        n165 = local write "%Open"(w539) -> ()
      }
    }
    n166 = And(x=w298, y=w313) -> (x .and. y?=w312:bool)
    n167 = And(x=w222, y=w308) -> (x .and. y?=w310:bool)
    n168 = And(x=w306, y=w308) -> (x .and. y?=w307:bool)
    n169 = Or(x=w307, y=w310) -> (x .or. y?=w309:bool)
    n170 = case shown="True" w312 {
      tunnel: w299 -> [_ w623]
      frame False {
      }
      frame True {
        n171 = Increment(x=w623) -> (x+1=w624:i32)
        n172 = Tick Count (ms)() -> (millisecond timer value=→"millisecond timer value":u32)
        n173 = property on="loop iter" class="DigNum (strict)"("Value"=w624) -> ()  [unwired: 2 in, 2 out]
      }
    }
    n174 = case shown="True" w309 {
      frame False {
      }
      frame True {
        n175 = Tick Count (ms)() -> (millisecond timer value=→"millisecond timer value 2":u32)
        n176 = property on="loop iter" class="DigNum (strict)"("Value"=2) -> ()  [unwired: 2 in, 2 out]
      }
    }
    n177 = Bundle("Oil Pump Speed Adjust"="Oil Pump Speed Adjust", "autotune? oil pump"="autotune? oil pump", "Fine slide in P 4"="Fine slide in P 4", "file for oil pump 3"="file for oil pump 3", "Accept Autotune Oil Pump"="Accept Autotune Oil Pump", "PID gains in oil pump"="PID gains in oil pump") -> (w163:T13)  [unwired: 1 in]
    n178 = call "CompressorSpeed.vi"("Controller Toggle P 2"="Controller Toggle P 6", "Compressor Input"=w209) -> ("output cluster"=w229:T14)  [unwired: 8 in, 1 out]
    n179 = Unbundle By Name(w229) -> ("output to slide"=→"Compressor Speed Output":dbl, "Controller Toggle P 2"=→"Controller Toggle P 5":bool)  [unwired: 2 out]
    n180 = local read "Units"() -> (w111:string)
    n181 = case shown="\"SI\", Default" w111 {
      tunnel: [w476 w478] -> w110
      tunnel: w109 -> [w475 w478]
      frame "SI", Default {
        n182 = node(w475) -> (w477:dbl[unit])
        n183 = node(w477) -> (w476:dbl)
      }
      frame "IP" {
      }
    }
    "Current Pdis" <- w110
    n184 = call "Oil Pump Speed.vi"("Controller Toggle P 2"="Controller Toggle P 8", "Compressor Input"=w163) -> ("output cluster"=w161:T14)  [unwired: 9 in]
    n185 = Unbundle By Name(w161) -> ("output to slide"=→"Oil Pump Output":dbl, "PID gains out"=→"PID gains out oil pump":T3, "tuning completed?"=→"tuning completed?":bool, "Controller Toggle P 2"=→"Controller Toggle Oil Pump":bool)
    n186 = Bundle("Coarse Water Adjust"="Coarse Water Adjust", "autotune? Coarse Water"="autotune? Coarse Water", "Fine slide in P 2"="Fine slide in P 2", "file for fine gas"="file for fine gas", "Accept Autotune Water"="Accept Autotune Water", "PID gains in Water Valve"="PID gains in Water Valve") -> (w200:T15)  [unwired: 1 in]
    n187 = Bundle("Fine Water Adjust"="Fine Water Adjust", "autotune? water pump 2"="autotune? water pump 2", "Fine slide in P 3"="Fine slide in P 3", "file for water pump 2"="file for water pump 2", "Accept Autotune Water Pump 2"="Accept Autotune Water Pump 2", "PID gains in water pump 2"="PID gains in water pump 2") -> (w193:T16)  [unwired: 1 in]
    n188 = local read "Units"() -> (w114:string)
    n189 = case shown="\"IP\"" w114 {
      tunnel: "Desired Pdis" -> [w480 w482]
      tunnel: [w479 w482] -> w112
      frame "SI", Default {
        n190 = node(w480) -> (w481:dbl[unit])
        n191 = node(w481) -> (w479:dbl)
      }
      frame "IP" {
      }
    }
    n192 = call "Water Valves.vi"("Condensing Press Threshold"="Condensing Press Threshold", "Current Pcond"=w109, "Desired Pcond"=w112, "Water Pump Input"=w193, "Reinitialize Controller"="Reinitialize Controller", "Controller Toggle P 2"="Controller Toggle P 4", "Water Valve Input"=w200) -> ("Water Control Out"=w139:T17)  [unwired: 4 in]
    n193 = Unbundle(w139) -> ("output to slide"=w126:dbl, "PID gains out"=→"PID gains out Coarse Water":T3, "tuning completed?"=→"tuning completed? Water Valve":bool, "output to slide"=w127:dbl, "PID gains out"=→"PID gains out (fine water)":T3, "tuning completed?"=→"tuning completed? Water Pump":bool, "Controller Toggle P 2"=w140:bool, w138:bool)
    "Water Valve Output" <- w126
    "Controller Toggle Water" <- w140
    "Water Pump Output" <- w127
    n194 = control-ref of="stop"() -> ()  [unwired: 1 out]
    n195 = case shown="True" w140 {
      tunnel: w138 -> [_ w525]
      tunnel: w127 -> [_ w524]
      tunnel: w126 -> [_ w523]
      frame False {
      }
      frame True {
        n196 = case shown="True" w525 {
          tunnel: w524 -> [_ w527]
          tunnel: w523 -> [w526 _]
          frame False {
            n197 = property on="Coarse Water Adjust" class="Slide (strict)"("Value"=w526) -> ()  [unwired: 2 in, 2 out]
          }
          frame True {
            n198 = property on="Fine Water Adjust" class="Slide (strict)"("Value"=w527) -> ()  [unwired: 2 in, 2 out]
          }
        }
      }
    }
    n199 = local read "Compressor VFD Output Frequency (Hz)"() -> (w93:dbl)
    n200 = control-ref of="Economizer\nFine Liquid Adjust"() -> (w377:refnum<vi>)
    n201 = control-ref of="Economizer\nLiquid Coarse Adjust"() -> (w381:refnum<vi>)
    n202 = control-ref of="Economizer Gas\n Coarse Adjust"() -> (w389:refnum<vi>)
    n203 = control-ref of="Economizer Gas\n Fine Adjust"() -> (w385:refnum<vi>)
    n204 = control-ref of="Medium Liquid Adjust"() -> (w434:refnum<vi>)
    n205 = control-ref of="Large Liquid Adjust  2"() -> (w428:refnum<vi>)
    n206 = control-ref of="Medium Gas Adjust"() -> (w416:refnum<vi>)
    n207 = control-ref of="Small Liquid Adjust"() -> (w440:refnum<vi>)
    n208 = control-ref of="Large Gas Adjust"() -> (w410:refnum<vi>)
    n209 = control-ref of="Small Gas Adjust"() -> (w422:refnum<vi>)
    n210 = Bundle("Economizer Gas\n Coarse Adjust"="Economizer Gas\n Coarse Adjust", "Accept Autotune Coarse"="Accept Autotune Coarse", "Economizer Gas\n Coarse Adjust"=w389, "Path 7"="Path 7", "Autotune Coarse"="Autotune Coarse", "PID gains in Coarse gas"="PID gains in Coarse gas") -> (w392:T18)  [unwired: 1 in]
    n211 = Bundle("Economizer Gas\n Fine Adjust"="Economizer Gas\n Fine Adjust", "Accept Autotune Fine"="Accept Autotune Fine", "Economizer Gas\n Fine Adjust"=w385, "Path 8"="Path 8", "Autotune Fine Gas"="Autotune Fine Gas", "PID gains in Fine Gas"="PID gains in Fine Gas") -> (w375:T19)  [unwired: 1 in]
    n212 = Bundle("Economizer\nLiquid Coarse Adjust"="Economizer\nLiquid Coarse Adjust", "Accept Autotune Coarse Liquid"="Accept Autotune Coarse Liquid", "Economizer\nLiquid Coarse Adjust"=w381, "Path 9"="Path 9", "Autotune CoarseLiquid"="Autotune CoarseLiquid", "PID gains in Coarse Liquid"="PID gains in Coarse Liquid") -> (w374:T20)  [unwired: 1 in]
    n213 = Bundle("Economizer\nFine Liquid Adjust"="Economizer\nFine Liquid Adjust", "Accept Autotune Fine Liquid"="Accept Autotune Fine Liquid", "Economizer\nFine Liquid Adjust"=w377, "Path 10"="Path 10", "Autotune Fine Liquid"="Autotune Fine Liquid", "PID gains in Fine Liquid"="PID gains in Fine Liquid") -> (w373:T21)  [unwired: 1 in]
    n214 = call "economizer exv valves.vi"("Coarse Gas Input Cluster"=w392, "Fine Gas Input Cluster"=w375, "Coarse Liq Input Cluster"=w374, "Fine Liq Input Cluster"=w373, "Controller Toggle P 2"="Controller Toggle P 2", "Reinitialize Controller P 2"=w372, "Economizer ?"="Economizer ?", "Current Intermediate T"="Current Intermediate T", "Desired Intermediate T"="Desired Intermediate T", "Desired Intermediate P"="Current Intermediate P", "Current Intermediate P"="Desired Intermediate P", "Controller Toggle T 2"="Controller Toggle T 2", "Reinitialize Controller T 2"=w371) -> ("Gas Valves Ouput"=w370:T22, "Liq Valves Ouput"=w369:T23)  [unwired: 13 in]
    n215 = Bundle("Large Gas Adjust"="Large Gas Adjust", "Autotune Large"="Autotune Large", "Path"="Path", "Large Gas Adjust"=w410, "Accept Autotune Large"="Accept Autotune Large", "PID gains in Large gas"="PID gains in Large gas") -> (w406:T24)  [unwired: 1 in]
    n216 = Bundle("Medium Gas Adjust"="Medium Gas Adjust", "Autotune Medium Gas"="Autotune Medium Gas", "Path 2"="Path 2", "Medium Gas Adjust"=w416, "Accept Autotune Medium"="Accept Autotune Medium", "PID gains in Medium Gas"="PID gains in Medium Gas") -> (w404:T25)  [unwired: 1 in]
    n217 = Bundle("Small Gas Adjust"="Small Gas Adjust", "Autotune Small"="Autotune Small", "Path 3"="Path 3", "Small Gas Adjust"=w422, "Accept Autotune Small"="Accept Autotune Small", "PID gains in Small Gas"="PID gains in Small Gas") -> (w405:T26)  [unwired: 1 in]
    n218 = Bundle("Large Liquid Adjust  2"="Large Liquid Adjust  2", "Autotune Large Liquid"="Autotune Large Liquid", "Path 4"="Path 4", "Large Liquid Adjust  2"=w428, "Accept Autotune Large  Liquid"="Accept Autotune Large  Liquid", "PID gains in Large Liquid"="PID gains in Large Liquid") -> (w403:T27)  [unwired: 1 in]
    n219 = Bundle("Medium Liquid Adjust"="Medium Liquid Adjust", "Autotune Medium Liquid"="Autotune Medium Liquid", "Path 5"="Path 5", "Medium Liquid Adjust"=w434, "Accept Autotune Medium Liquid"="Accept Autotune Medium Liquid", "PID gains in Medium Liquid"="PID gains in Medium Liquid") -> (w402:T28)  [unwired: 1 in]
    n220 = Bundle("Small Liquid Adjust"="Small Liquid Adjust", "Autotune Small Liquid"="Autotune Small Liquid", "Path 6"="Path 6", "Small Liquid Adjust"=w440, "Accept Autotune Small Liquid"="Accept Autotune Small Liquid", "PID gains in Small Liquid"="PID gains in Small Liquid") -> (w401:T29)  [unwired: 1 in]
    n221 = case shown="\"IP\"" "Units" {
      tunnel: "Desired Tsuc" -> [w486 w489]
      tunnel: [w486 w488] -> w117
      tunnel: "Desired Psuc" -> [w484 w487]
      tunnel: [w483 w487] -> w115
      frame "SI", Default {
        n222 = node(w484) -> (w485:dbl[unit])
        n223 = node(w485) -> (w483:dbl)
      }
      frame "IP" {
        n224 = node(w489) -> (w490:dbl[unit])
        n225 = node(w490) -> (w488:dbl)
      }
    }
    n226 = Unbundle(w369) -> ("Liquid\n Fine Position"=→"Economizer\nFine Liquid Position":dbl, "PID gains out fine liq"=→"PID gains out Fine Liquid":T3, "tuning completed? fine liq"=→"tuning completed? Fine Liquid":bool, "Liquid\n Coarse Position"=→"Economizer\nLiquid Coarse Position":dbl, "PID gains out coarse liq"=→"PID gains out Coarse Liquid":T3, "tuning completed? coarse liq"=→"tuning completed? Coarse Liquid":bool, "T Indicator"=→"Controller Toggle T 3":bool)
    n227 = Unbundle(w370) -> ("Hot Gas Bypass\n Fine Position"=→"Economizer Gas\n Fine Position":dbl, "PID gains out fine gas"=→"PID gains out Fine Gas":T3, "tuning completed? fine gas"=→"tuning completed? Fine Gas":bool, "Hot Gas Bypass\n Coarse Position"=→"Economizer Gas\n Coarse Position":dbl, "PID gains out coarse gas"=→"PID gains out Coarse Gas":T3, "tuning completed? coarse gas"=→"tuning completed? Coarse Gas":bool, "P Indicator"=→"Controller Toggle P 3":bool)
    n228 = call "exv valves.vi"("Large Gas Cluster"=w406, "Medium Gas Cluster"=w404, "Small Gas Cluster"=w405, "Large Liquid Cluster"=w403, "Medium Liquid Cluster"=w402, "Small Liquid Cluster"=w401, "Tonnage"=w282, "Desired Psuc"=w115, "Reinitialize Controller P"=w463, "Controller Toggle P"="?", "Tonnage Threshold"=w461, "Desired Tsuc"=w117, "Delta P Threshold"=w459, "Current Psuc"=w160, "Delta T Threshold"=w460, "Current Tsuc"=w106, "Reinitialize Controller T"=w462, "Controller Toggle T"="?") -> ("Gas Valves Output"=w137:T30, "Liquid Valves Output"=w136:T31)  [unwired: 8 in]
    n229 = case shown="True" "Are the values not stupid numbers anymore?" {
      frame False {
      }
      frame True {
        n230 = local read "Pdis2"() -> (w531:dbl)
        n231 = local read "Pdis"() -> (w535:dbl)
        n232 = Greater Or Equal?(x=w535, y=455.0) -> (x >= y?=w533:bool)
        n233 = Greater Or Equal?(x=w531, y=455.0) -> (x >= y?=w530:bool)
        n234 = Or(x=w533, y=w530) -> (x .or. y?=w529:bool)
        n235 = Or(x="?", y=w529) -> (x .or. y?=w536:bool)
        n236 = shared-variable ".\\Untitled Library 2.lvlib\\Stop1"(w536) -> ()  [unwired: 1 in, 1 out]
      }
    }
    n237 = Unbundle(w137) -> ("output to slide"=w128:dbl, "PID gains out"=→"PID gains out Large Gas":T3, "tuning completed?"=→"tuning completed? Large Gas":bool, "output to slide"=w123:dbl, "PID gains out"=→"PID gains out Medium Gas":T3, "tuning completed?"=→"tuning completed? Medium Gas":bool, "output to slide"=w122:dbl, "PID gains out"=→"PID gains out Small Gas":T3, "tuning completed?"=→"tuning completed? Small Gas":bool, "Controller Toggle P"=w131:bool, w130:bool, w129:bool)
    "Output Large Gas" <- w128
    "Output Medium Gas" <- w123
    "Output Small Gas" <- w122
    "Controller Toggle P" <- w131
    n238 = Unbundle(w136) -> ("output to slide"=w132:dbl, "PID gains out"=→"PID gains out Large Liquid":T3, "tuning completed?"=→"tuning completed? Large Liq":bool, "output to slide"=w121:dbl, "PID gains out"=→"PID gains out Medium Liquid":T3, "tuning completed?"=→"tuning completed? Medium Liq":bool, "output to slide"=w120:dbl, "PID gains out"=→"PID gains out Small Liquid":T3, "tuning completed?"=→"tuning completed? Small Liq":bool, "Controller Toggle T"=w135:bool, w134:bool, w133:bool)
    "Output Large Liq" <- w132
    "Output Medium Liq" <- w121
    "Output Small Liq" <- w120
    "Controller Toggle T" <- w135
    n239 = Build Array(w126, w127, w123, w122, w121, w120, w93) -> (w125:dbl[])
    n240 = Bundle By Name(cluster=w333, "RTDs"=w464, "Thermocouples"=w466, "Pressure Transducers"=w465, "Mass Flow Meters"=w446, "Barometer"=w349, "Accelerometer"=w328, "Power"=w188, "Valve Positions"=w125) -> (w124:T1)
    n241 = shared-variable "NI-cRIO-9035-01CA85F4\\Untitled Library 4.lvlib\\output cluster"(w124) -> ()  [unwired: 1 in, 1 out]
    n242 = case shown="True" w135 {
      tunnel: w134 -> [_ w512]
      tunnel: w133 -> [_ w511]
      tunnel: w120 -> [_ w510]
      tunnel: w121 -> [_ w509]
      tunnel: w121 -> [_ w508]
      tunnel: w132 -> [_ w507]
      frame False {
      }
      frame True {
        n243 = case shown="True" w512 {
          tunnel: w511 -> [w515 w520]
          tunnel: w510 -> [_ w519]
          tunnel: w509 -> [_ w518]
          tunnel: w508 -> [w514 _]
          tunnel: w507 -> [w513 _]
          frame False {
            n244 = case shown="True" w515 {
              tunnel: w514 -> [_ w517]
              tunnel: w513 -> [w516 _]
              frame False {
                n245 = property on="Large Liquid Adjust  2" class="Slide (strict)"("Value"=w516) -> ()  [unwired: 2 in, 2 out]
              }
              frame True {
                n246 = property on="Medium Liquid Adjust" class="Slide (strict)"("Value"=w517) -> ()  [unwired: 2 in, 2 out]
              }
            }
          }
          frame True {
            n247 = case shown="True" w520 {
              tunnel: w519 -> [_ w522]
              tunnel: w518 -> [w521 _]
              frame False {
                n248 = property on="Medium Liquid Adjust" class="Slide (strict)"("Value"=w521) -> ()  [unwired: 2 in, 2 out]
              }
              frame True {
                n249 = property on="Small Liquid Adjust" class="Slide (strict)"("Value"=w522) -> ()  [unwired: 2 in, 2 out]
              }
            }
          }
        }
      }
    }
    n250 = case shown="True" w131 {
      tunnel: w130 -> [_ w496]
      tunnel: w122 -> [_ w495]
      tunnel: w123 -> [_ w494]
      tunnel: w129 -> [_ w493]
      tunnel: w123 -> [_ w492]
      tunnel: w128 -> [_ w491]
      frame False {
      }
      frame True {
        n251 = case shown="True" w496 {
          tunnel: w495 -> [_ w504]
          tunnel: w494 -> [_ w503]
          tunnel: w493 -> [w499 w502]
          tunnel: w492 -> [w498 _]
          tunnel: w491 -> [w497 _]
          frame False {
            n252 = case shown="False" w499 {
              tunnel: w498 -> [_ w501]
              tunnel: w497 -> [w500 _]
              frame False {
                n253 = property on="Large Gas Adjust" class="Slide (strict)"("Value"=w500) -> ()  [unwired: 2 in, 2 out]
              }
              frame True {
                n254 = property on="Medium Gas Adjust" class="Slide (strict)"("Value"=w501) -> ()  [unwired: 2 in, 2 out]
              }
            }
          }
          frame True {
            n255 = case shown="False" w502 {
              tunnel: w504 -> [_ w506]
              tunnel: w503 -> [w505 _]
              frame False {
                n256 = property on="Medium Gas Adjust" class="Slide (strict)"("Value"=w505) -> ()  [unwired: 2 in, 2 out]
              }
              frame True {
                n257 = property on="Small Gas Adjust" class="Slide (strict)"("Value"=w506) -> ()  [unwired: 2 in, 2 out]
              }
            }
          }
        }
      }
    }
    n258 = control-ref of="Data Rate"() -> (w342:refnum<vi>)
    n259 = call "Accelerometer plot.vi"("Refnum in"=w346, "Ring Refnum"=w342, "Host Loop update rate (ms)"="Host Loop update rate (ms)", "stop"="stop", "error in (no error)"=w345) -> ("size(s)"=→"size(s)":i32, "Spool x acceleration"=w97:dbl[][], "acceleration v time"=→"acceleration v time":waveform(dbl)[], "rotational speed (rpm)"=→"rotational speed (rpm)":dbl, "Open Loop"=→"Open Loop":bool[], "Elements Remaining"=→"Elements Remaining":u32, "Short Circuit"=→"Short Circuit":bool[], "Waveform Graph"=→"Waveform Graph":waveform(dbl)[], "Spool y acceleration"=w103:dbl[][], "Array"=w180:dbl[][], "Refnum out"=w344:refnum<k20>, 21:"error out"=w343:errorcluster, "magnitudes"=→"magnitudes":cluster{"f0":dbl, "df":dbl, "magnitude":dbl[]}[], "Data FIFO Full"=→"Data FIFO Full":bool, "result"=→"result":bool, 27:"error out"=w335:errorcluster)  [unwired: 6 in, 1 out]
    n260 = Index Array(array=w180, index (row)=0, index (col)=0 ("disabled index (col)")) -> (element=→"Compressor Speed (Hz)":dbl)
    n261 = Index Array(array=w97, index (row)=0, index (col)=0 ("disabled index (col)")) -> (element=→"Spool x acceleration (Hz)":dbl)
    n262 = Index Array(array=w103, index (row)=0, index (col)=0 ("disabled index (col)")) -> (element=→"Spool y acceleration (Hz)":dbl)
    n263 = shared-variable ".\\Untitled Library 2.lvlib\\Stop1"() -> (w191:bool)  [unwired: 1 in, 1 out]
    n264 = node-c288() -> ()  [unwired: 1 in, 1 out]
  }
  "FPGA Error Out" <- w65
  "FPGA error out" <- w13
  n265 = xnode "Close FPGA VI Reference"("FPGA VI Reference In"=w12) -> ("error out"=→"Host error out 3":errorcluster)  [unwired: 1 in]
  n266 = node-c288(w4) -> ()  [unwired: 1 out]
  n267 = xnode "Close FPGA VI Reference"("FPGA VI Reference In"=w26, "error in"=w67) -> ("error out"=→"Host error out":errorcluster)
  "loop iter" <- w10
  "loop iter 2" <- w10
  "loop iter 3" <- w9
  "loop iter 4" <- w9
